vi "AWG Initialize.vi"(8 "error in (no error)":errorcluster, 9 "Reset (True)":bool=TRUE, 10 "ID Query (True)":bool=TRUE, 11 "awg session in":T1={"type"=enum."Agilent 331xxA to 332xxA", "VISA"="", "enable 10MHz ref"=FALSE, "cmi ckd2"={"VISA"="", "clock source"=enum."Auto", "manual ref clk"=FALSE, "ref clock [Hz]"=0.0, "div mode"=enum."Set divisor directly"}, "cmi sync v3"={"VISA"="", "baud rate [bd/s]"=115200, "source"=enum."Auto", "hv range"=enum."1kV", "fsrc is fixed"=FALSE, "fsrc [Hz]"=10000000.0, "freq integ [s]"=1.0, "freq filter"=5, "trig level"=enum."TTL 5V", "chn1 mode"=enum."Source divider", "chn1 level"=enum."Positive 5V", "chn2 mode"=enum."Source divider", "chn2 level"=enum."Positive 5V", "chn2 div"=1, "chn3 mode"=enum."Chn 1 Active", "chn3 level"=enum."Positive 5V", "chn1 div entry"=enum."Calculate nearest divisor from measured fx", "chn1 dev limit [%]"=1.0, "chn1 check dev"=FALSE}, "trigger"={"source"=enum."Immediate", "level [V]"=0.0, "coupling"=enum."DC", "slope"=enum."POS"}, "HMF2500 cfg"={"Baud Rate"=9600, "Parity"=0, "Data Bits"=8, "Flow Control"=4}} {"HMF2500 cfg"."Flow Control" items=["None", "XON/XOFF", "RTS/CTS", "XON/XOFF & RTS/CTS", "DTR/DSR", "XON/XOFF & DTR/DSR"]; "HMF2500 cfg"."Data Bits" items=["7"=7, "8"=8]; "HMF2500 cfg"."Parity" items=["None", "Odd", "Even", "Mark", "Space"]; "HMF2500 cfg"."Baud Rate" items=["300"=300, "600"=600, "1200"=1200, "2400"=2400, "4800"=4800, "9600"=9600, "19200"=19200]; "cmi sync v3"."chn2 div" min=1 max=100000000 step=1; "cmi sync v3"."fsrc [Hz]" format="%_8p"}) -> (0 "error out":errorcluster, 2 "idn string":string, 3 "awg session out":T1={"type"=enum."Agilent 331xxA to 332xxA", "VISA"="", "enable 10MHz ref"=FALSE, "cmi ckd2"={"VISA"="", "clock source"=enum."Auto", "manual ref clk"=FALSE, "ref clock [Hz]"=0.0, "div mode"=enum."Set divisor directly"}, "cmi sync v3"={"VISA"="", "baud rate [bd/s]"=115200, "source"=enum."Auto", "hv range"=enum."1kV", "fsrc is fixed"=FALSE, "fsrc [Hz]"=10000000.0, "freq integ [s]"=1.0, "freq filter"=5, "trig level"=enum."TTL 5V", "chn1 mode"=enum."Source divider", "chn1 level"=enum."Positive 5V", "chn2 mode"=enum."Source divider", "chn2 level"=enum."Positive 5V", "chn2 div"=1, "chn3 mode"=enum."Chn 1 Active", "chn3 level"=enum."Positive 5V", "chn1 div entry"=enum."Calculate nearest divisor from measured fx", "chn1 dev limit [%]"=1.0, "chn1 check dev"=FALSE}, "trigger"={"source"=enum."Immediate", "level [V]"=0.0, "coupling"=enum."DC", "slope"=enum."POS"}, "HMF2500 cfg"={"Baud Rate"=9600, "Parity"=0, "Data Bits"=8, "Flow Control"=4}} {"HMF2500 cfg"."Flow Control" items=["None", "XON/XOFF", "RTS/CTS", "XON/XOFF & RTS/CTS", "DTR/DSR", "XON/XOFF & DTR/DSR"]; "HMF2500 cfg"."Data Bits" items=["7"=7, "8"=8]; "HMF2500 cfg"."Parity" items=["None", "Odd", "Even", "Mark", "Space"]; "HMF2500 cfg"."Baud Rate" items=["300"=300, "600"=600, "1200"=1200, "2400"=2400, "4800"=4800, "9600"=9600, "19200"=19200]; "cmi sync v3"."chn2 div" min=1 max=100000000 step=1; "cmi sync v3"."fsrc [Hz]" format="%_8p"})   [LabVIEW 2020, in "AWG.lvlib"]
doc: "AWG wrapper: initialize function generator."
uses:
  AWG.lvlib
  AWG Session.ctl
  AWG Type.ctl
  CMI Clock Divider v2/CMI ckd2 Session.ctl
  CMI Clock Divider v2/CMI ckd2 Source Mode.ctl
  CMI Clock Divider v2/CMI ckd2 Divisor Mode.ctl
  CMI Sync V3/CMI Sync V3 session.ctl
  CMI Sync V3/Configure/CMI Sync V3 Reference Clock Source.ctl
  CMI Sync V3/Configure/CMI Sync V3 HV input Range.ctl
  CMI Sync V3/Configure/CMI Sync V3 Trigger Input Level.ctl
  CMI Sync V3/Configure/CMI Sync V3 Channel 1 Mode.ctl
  CMI Sync V3/Configure/CMI Sync V3 Channel Output Levels.ctl
  CMI Sync V3/Configure/CMI Sync V3 Channel 2 Mode.ctl
  CMI Sync V3/Configure/CMI Sync V3 Channel 3 Mode.ctl
  CMI Sync V3/Configure/CMI Sync V3 Channel 1 Divisor Entry Mode.ctl
  externals needed for AWG/ADC Trig Config.ctl
  externals needed for AWG/ADC Trig Mode Source.ctl
  externals needed for AWG/ADC Trig Coupling.ctl
  externals needed for AWG/ADC Trig Slope.ctl
  RaS HMF2500/HMF2500 Config.ctl
  Agilent 33XXX Series/Agilent 33XXX Series.lvlib
  Agilent 3352X Series/Agilent 3352X Series.lvlib
  AFG3000/Tektronix AFG 3000 Series.lvlib
  CMI Sync V3/CMI Sync Unit V3.lvlib
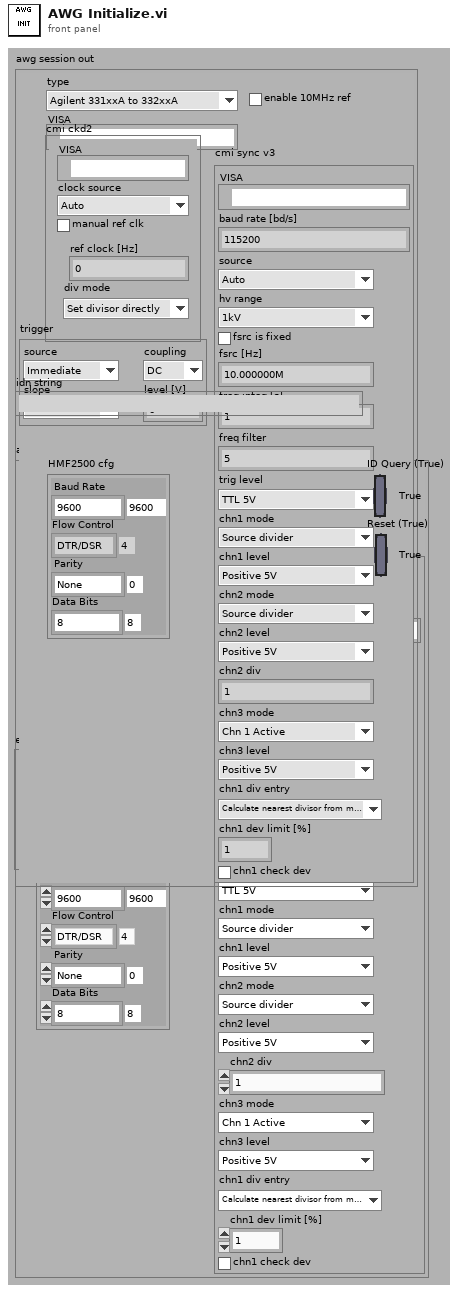
[diagram p1: front panel]
types:
  T1 = typedef "AWG.lvlib/AWG Session.ctl" = cluster{"type":T2, "VISA":refnum<visa-resource-name>, "enable 10MHz ref":bool, "cmi ckd2":T3, "cmi sync v3":T6, "trigger":T15, "HMF2500 cfg":T19}
  T2 = typedef "AWG.lvlib/AWG Type.ctl" = enum16{"Agilent 331xxA to 332xxA", "Agilent 335xxA to 336xxA", "Tektronix AFG3101C", "R&S HMF25xx", "CMI Clock Divider v2", "CMI Sync Unit V3", "dummy"}
  T3 = typedef "AWG.lvlib/CMI ckd2 Session.ctl" = cluster{"VISA":refnum<visa-resource-name>, "clock source":T4, "manual ref clk":bool, "ref clock [Hz]":dbl, "div mode":T5}
  T4 = typedef "AWG.lvlib/CMI ckd2 Source Mode.ctl" = enum16{"Auto", "LF clock", "HF clock", "Internal"}
  T5 = typedef "AWG.lvlib/CMI ckd2 Divisor Mode.ctl" = enum16{"Set divisor directly", "Set divisor by frequency"}
  T6 = typedef "AWG.lvlib/CMI Sync Unit V3.lvlib/CMI Sync V3 session.ctl" = cluster{"VISA":refnum<visa-resource-name>, "baud rate [bd/s]":i32, "source":T7, "hv range":T8, "fsrc is fixed":bool, "fsrc [Hz]":dbl, "freq integ [s]":dbl, "freq filter":i32, "trig level":T9, "chn1 mode":T10, "chn1 level":T11, "chn2 mode":T12, "chn2 level":T11, "chn2 div":i32, "chn3 mode":T13, "chn3 level":T11, "chn1 div entry":T14, "chn1 dev limit [%]":dbl, "chn1 check dev":bool}
  T7 = typedef "AWG.lvlib/CMI Sync Unit V3.lvlib/CMI Sync V3 Reference Clock Source.ctl" = enum16{"Auto", "Internal", "Logic", "Sine", "HV"}
  T8 = typedef "AWG.lvlib/CMI Sync Unit V3.lvlib/CMI Sync V3 HV input Range.ctl" = enum16{"10V", "60V", "250V", "1kV"}
  T9 = typedef "AWG.lvlib/CMI Sync Unit V3.lvlib/CMI Sync V3 Trigger Input Level.ctl" = enum16{"LVCMOS 3V3", "TTL 5V"}
  T10 = typedef "AWG.lvlib/CMI Sync Unit V3.lvlib/CMI Sync V3 Channel 1 Mode.ctl" = enum16{"Source divider", "DDS absolute", "DDS ratio", "DDS ratio M/N"}
  T11 = typedef "AWG.lvlib/CMI Sync Unit V3.lvlib/CMI Sync V3 Channel Output Levels.ctl" = enum16{"Positive 3V3", "Negative 3V3", "Positive 5V", "Negative 5V"}
  T12 = typedef "AWG.lvlib/CMI Sync Unit V3.lvlib/CMI Sync V3 Channel 2 Mode.ctl" = enum16{"Source divider", "Chn 1 divide"}
  T13 = typedef "AWG.lvlib/CMI Sync Unit V3.lvlib/CMI Sync V3 Channel 3 Mode.ctl" = enum16{"Chn 1 Active", "Chn 2 Active", "Chn 1 Trigger", "Chn 2 Trigger", "Gate", "PPS", "10MHz"}
  T14 = typedef "AWG.lvlib/CMI Sync Unit V3.lvlib/CMI Sync V3 Channel 1 Divisor Entry Mode.ctl" = enum16{"Set divisor directly", "Calculate nearest divisor from measured fx"}
  T15 = typedef "ADC Trig Config.ctl" = cluster{"source":T16, "level [V]":dbl, "coupling":T17, "slope":T18}
  T16 = typedef "ADC Trig Mode Source.ctl" = enum16{"Immediate", "External", "Level"}
  T17 = typedef "ADC Trig Coupling.ctl" = enum16{"DC", "AC"}
  T18 = typedef "ADC Trig Slope.ctl" = enum16{"POS", "NEG"}
  T19 = typedef "AWG.lvlib/HMF2500 Config.ctl" = cluster{"Baud Rate":u32, "Parity":u16, "Data Bits":u16, "Flow Control":u16}
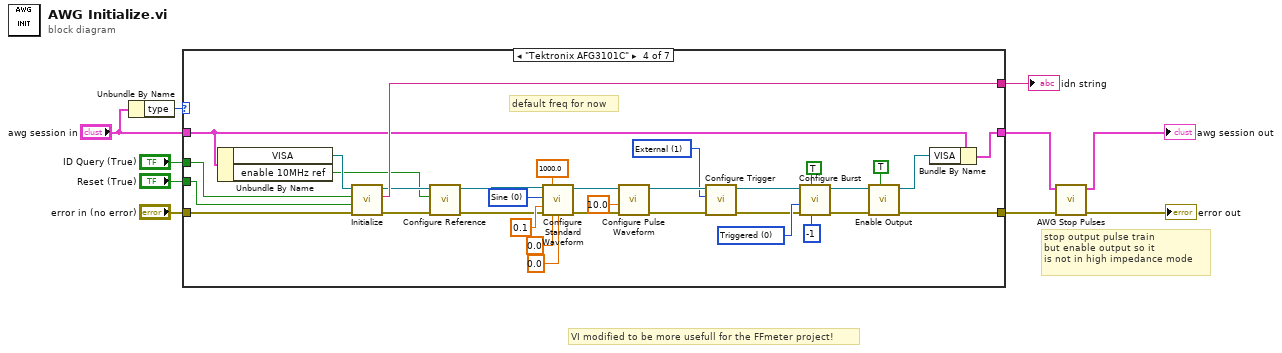
[diagram p0: block diagram]
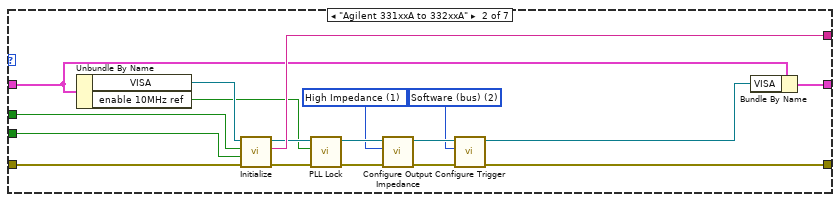
[diagram p3: hidden frame]
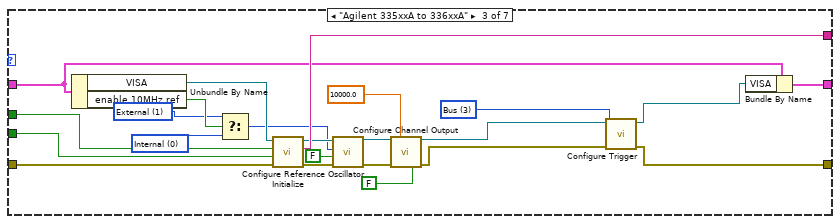
[diagram p4: hidden frame]
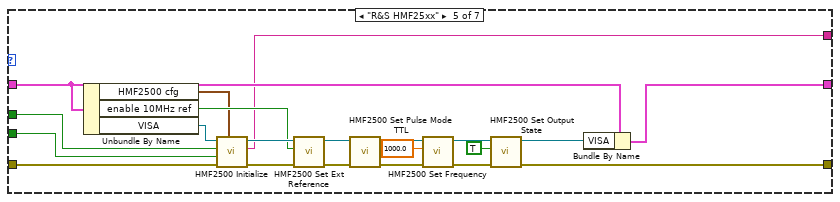
[diagram p5: hidden frame]
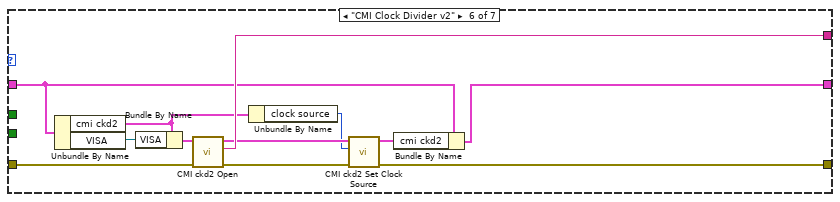
[diagram p6: hidden frame]
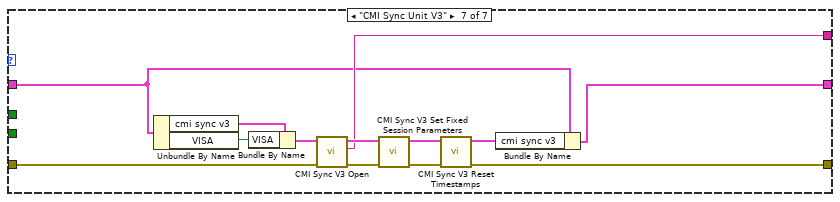
[diagram p7: hidden frame]
diagram:
  # "VI modified to be more usefull for the FFmeter project!"
  # "stop output pulse train\nbut enable output so it \nis not in high impedance mode"
  n1 = Unbundle By Name("awg session in") -> ("type"=w10:T2)
  n2 = case shown="\"Tektronix AFG3101C\"" w10 {
    tunnel: "error in (no error)" -> [w12 w30 w53 w86 w107 w119 w132]
    tunnel: [_ w29 w52 w82 w87 w116 w129] -> w8
    tunnel: [w12 w13 w32 w69 w90 w111 w123] -> w4
    tunnel: "awg session in" -> [w11 w26 w50 w68 w92 w110 w128]
    tunnel: [w11 w27 w49 w66 w89 w108 w127] -> w2
    tunnel: "ID Query (True)" -> [_ w25 w45 w84 w105 _ _]
    tunnel: "Reset (True)" -> [_ w24 w44 w85 w104 _ _]
    frame Default {
    }
    frame "Agilent 331xxA to 332xxA" {
      w15 = u16 2 items=["Internal", "External", "Software (bus)"] ("Trigger Source (0: Internal)")
      w18 = u16 1 items=["50 Ohms", "High Impedance", "User Defined"] ("Impedance (0: 50 Ohms)")
      n3 = Unbundle By Name(w26) -> ("VISA"=w28:refnum<visa-resource-name>, "enable 10MHz ref"=w21:bool)
      n4 = call "Initialize.vi"("error in (no error)"=w30, "Reset (True)"=w24, "ID Query (True)"=w25, "VISA resource name"=w28) -> ("error out"=w23:errorcluster, "idn string"=w29:string, "VISA resource name out"=w22:refnum<visa-resource-name>)  [unwired: 5 in]
      n5 = call "PLL Lock.vi"("error in (no error)"=w23, "PLL lock  (T: Enable)"=w21, "VISA resource name"=w22) -> ("error out"=w20:errorcluster, "VISA resource name out"=w19:refnum<visa-resource-name>)  [unwired: 7 in]
      n6 = call "Configure Output Impedance.vi"("error in (no error)"=w20, "Impedance (0: 50 Ohms)"=w18, "VISA resource name"=w19) -> ("error out"=w17:errorcluster, "VISA resource name out"=w16:refnum<visa-resource-name>)  [unwired: 7 in]
      n7 = call "Configure Trigger.vi"("error in (no error)"=w17, "Trigger Source (0: Internal)"=w15, "VISA resource name"=w16) -> ("error out"=w13:errorcluster, "VISA resource name out"=w14:refnum<visa-resource-name>)  [unwired: 7 in]
      n8 = Bundle By Name(cluster=w26, "VISA"=w14) -> (w27:T1)
    }
    frame "Agilent 335xxA to 336xxA" {
      w31 = 3 items=["Immediate", "External", "Timer", "Bus"] ("Trigger Source (0: Immediate)")
      w37 = 1 items=["Internal", "External"] ("Source (0: Internal)")
      w36 = 0 items=["Internal", "External"] ("Source (0: Internal)")
      n9 = Unbundle By Name(w50) -> ("VISA"=w51:refnum<visa-resource-name>, "enable 10MHz ref"=w46:bool)
      n10 = Select(t=w37, s=w46, f=w36) -> (s? t:f=w38:i32)
      n11 = call "Initialize.vi"("error in (no error)"=w53, "Reset (Enable)"=w44, "ID Query (Enable)"=w45, "VISA resource name"=w51) -> ("error out"=w47:errorcluster, "idn string"=w52:string, "VISA resource name out"=w48:refnum<visa-resource-name>)  [unwired: 5 in]
      n12 = call "Configure Reference Oscillator.vi"("error in (no error)"=w47, "Source Auto Selection(T: Enable)"=FALSE, "Source (0: Internal)"=w38, "VISA resource name"=w48) -> ("error out"=w43:errorcluster, "VISA resource name out"=w42:refnum<visa-resource-name>)  [unwired: 6 in]
      n13 = call "Configure Channel Output.vi"("VISA resource name"=w42, "Output Impedance (50 Ohm)"=10000.0, "error in (no error)"=w43, "Enable Voltage Limit (T: Enable)"=FALSE) -> ("VISA resource name out"=w35:refnum<visa-resource-name>, "error out"=w33:errorcluster)  [unwired: 10 in]
      n14 = call "Configure Trigger.vi"("error in (no error)"=w33, "Trigger Source (0: Immediate)"=w31, "VISA resource name"=w35) -> ("error out"=w32:errorcluster, "VISA resource name out"=w34:refnum<visa-resource-name>)  [unwired: 7 in]
      n15 = Bundle By Name(cluster=w50, "VISA"=w34) -> (w49:T1)
    }
    frame "Tektronix AFG3101C" {
      w54 = u16 1 items=["Internal"=3, "External"=1] ("Trigger Source (3:Internal)")
      w73 = u16 0 items=["Triggered", "Gated"] ("Burst Mode (0: Triggered)")
      w78 = u16 0 items=["Sine", "Square", "Pulse", "Ramp", "Noise", "DC", "Sin(x)/x", "Gaussian", "Lorentz", "Exponential Rise", "Exponential Decay", "Haversine"] ("Waveform Function (0: Sine)")
      # "default freq for now"
      n16 = Unbundle By Name(w68) -> ("VISA"=w83:refnum<visa-resource-name>, "enable 10MHz ref"=w60:bool)
      n17 = call "Initialize.vi"("error in (no error)"=w86, "Reset (True)"=w85, "ID Query (True)"=w84, "VISA resource name"=w83) -> ("error out"=w64:errorcluster, "idn string"=w82:string, "VISA resource name out"=w63:refnum<visa-resource-name>)  [unwired: 5 in]
      n18 = call "Configure Reference.vi"("error in (no error)"=w64, "external clock"=w60, "VISA resource name"=w63) -> ("error out"=w62:errorcluster, "VISA resource name out"=w61:refnum<visa-resource-name>)  [unwired: 7 in]
      n19 = call "Configure Standard Waveform.vi"("VISA resource name"=w61, "Frequency (1000 Hz)"=1000.0, "Waveform Function (0: Sine)"=w78, "Amplitude (1 Vpp)"=0.1, "error in (no error)"=w62, "DC Offset (0.00 V)"=0.0, "Phase Level (-1)"=0.0) -> ("VISA resource name out"=w75:refnum<visa-resource-name>, "error out"=w76:errorcluster)  [unwired: 7 in]
      n20 = call "Configure Pulse Waveform.vi"("error in (no error)"=w76, "Duty Cycle (50%)"=10.0, "VISA resource name"=w75) -> ("error out"=w58:errorcluster, "VISA resource name out"=w55:refnum<visa-resource-name>)  [unwired: 7 in]
      n21 = call "Configure Trigger.vi"("error in (no error)"=w58, "Trigger Source (3:Internal)"=w54, "VISA resource name"=w55) -> ("error out"=w57:errorcluster, "VISA resource name out"=w56:refnum<visa-resource-name>)  [unwired: 7 in]
      n22 = call "Configure Burst.vi"("Burst Count (5)"=-1, "Enable Burst (T: Enable)"=TRUE, "error in (no error)"=w57, "Burst Mode (0: Triggered)"=w73, "VISA resource name"=w56) -> ("error out"=w71:errorcluster, "VISA resource name out"=w70:refnum<visa-resource-name>)  [unwired: 5 in]
      n23 = call "Enable Output.vi"("Enable Output (T: Enable)"=TRUE, "error in (no error)"=w71, "VISA resource name"=w70) -> ("error out"=w69:errorcluster, "VISA resource name out"=w67:refnum<visa-resource-name>)  [unwired: 7 in]
      n24 = Bundle By Name(cluster=w68, "VISA"=w67) -> (w66:T1)
    }
    frame "R&S HMF25xx" {
      n25 = Unbundle By Name(w92) -> ("HMF2500 cfg"=w88:T19, "enable 10MHz ref"=w101:bool, "VISA"=w106:refnum<visa-resource-name>)
      n26 = call "HMF2500 Initialize.vi"("Serial Configuration"=w88, "error in (no error)"=w107, "Reset (True)"=w104, "ID Query (True)"=w105, "VISA resource name"=w106) -> ("error out"=w103:errorcluster, "idn string"=w87:string, "VISA resource name out"=w102:refnum<visa-resource-name>)  [unwired: 4 in]
      n27 = call "HMF2500 Set Ext Reference.vi"("error in (no error)"=w103, "Uset Ext Ref Clock (False)"=w101, "VISA in"=w102) -> ("error out"=w100:errorcluster, "VISA out"=w99:refnum<visa-resource-name>)  [unwired: 7 in]
      n28 = call "HMF2500 Set Pulse Mode TTL.vi"("error in (no error)"=w100, "VISA in"=w99) -> ("error out"=w97:errorcluster, "VISA out"=w94:refnum<visa-resource-name>)  [unwired: 8 in]
      n29 = call "HMF2500 Set Frequency.vi"("error in (no error)"=w97, "frequency [Hz] (1000)"=1000.0, "VISA in"=w94) -> ("error out"=w96:errorcluster, "VISA out"=w95:refnum<visa-resource-name>)  [unwired: 7 in]
      n30 = call "HMF2500 Set Output State.vi"("error in (no error)"=w96, "Enabled (False)"=TRUE, "VISA in"=w95) -> ("error out"=w90:errorcluster, "VISA out"=w91:refnum<visa-resource-name>)  [unwired: 7 in]
      n31 = Bundle By Name(cluster=w92, "VISA"=w91) -> (w89:T1)
    }
    frame "CMI Clock Divider v2" {
      n32 = Unbundle By Name(w110) -> ("cmi ckd2"=w113:T3, "VISA"=w118:refnum<visa-resource-name>)
      n33 = Bundle By Name(cluster=w113, "VISA"=w118) -> (w117:T3)
      n34 = call "CMI ckd2 Open.vi"("error in"=w119, "session"=w117) -> ("error out"=w115:errorcluster, "read buffer"=w116:string, "session out"=w114:T3)  [unwired: 7 in]
      n35 = Unbundle By Name(w113) -> ("clock source"=w112:T4)
      n36 = call "CMI ckd2 Set Clock Source.vi"("error in"=w115, "clock source (auto)"=w112, "session"=w114) -> ("error out"=w111:errorcluster, "session out"=w109:T3)  [unwired: 7 in]
      n37 = Bundle By Name(cluster=w110, "cmi ckd2"=w109) -> (w108:T1)
    }
    frame "CMI Sync Unit V3" {
      n38 = Unbundle By Name(w128) -> ("cmi sync v3"=w122:T6, "VISA"=w121:refnum<visa-resource-name>)
      n39 = Bundle By Name(cluster=w122, "VISA"=w121) -> (w120:T6)
      n40 = call "CMI Sync V3 Open.vi"("error in"=w132, "session in"=w120) -> ("error out"=w131:errorcluster, "identification string"=w129:string, "session out"=w130:T6)  [unwired: 7 in]
      n41 = call "CMI Sync V3 Set Fixed Session Parameters.vi"("error in"=w131, "session in"=w130) -> ("error out"=w126:errorcluster, "session out"=w125:T6)  [unwired: 8 in]
      n42 = call "CMI Sync V3 Reset Timestamps.vi"("error in"=w126, "session in"=w125) -> ("error out"=w123:errorcluster, "session out"=w124:T6)  [unwired: 8 in]
      n43 = Bundle By Name(cluster=w128, "cmi sync v3"=w124) -> (w127:T1)
    }
  }
  "idn string" <- w8
  n44 = call "AWG Stop Pulses.vi"("error in (no error)"=w4, "awg session in"=w2) -> ("error out"=→"error out":errorcluster, "awg session out"=→"awg session out":T1)  [unwired: 8 in]
